vi "Cal_MinimumTriggerStep_from_SweepSpeed.vi"(8 "error in (no error)":errorcluster, 10 "speed":dbl, 11 ".NET Reference in":refnum<k24>) -> (0 "error out":errorcluster, 2 "triggerstep out":dbl, 3 "Reference out":refnum<k24>)   [LabVIEW 2017]
uses:
  LV_IL_Sample/DLL/InstrumentDLL.dll
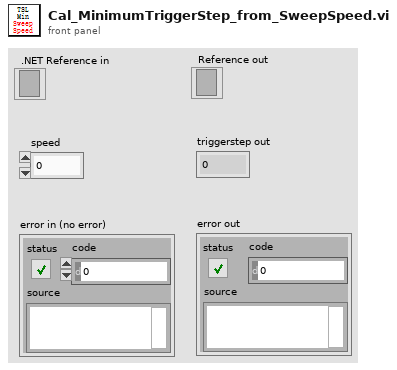
[diagram p1: front panel]
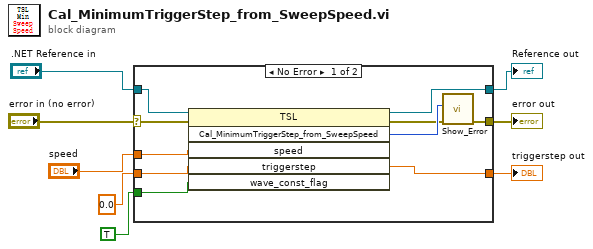
[diagram p0: block diagram]
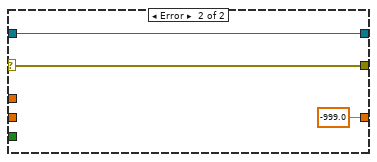
[diagram p2: hidden frame]
diagram:
  n1 = case shown="No Error" "error in (no error)" {
    selector: "error in (no error)" -> [w9 w19]
    tunnel: "speed" -> [w18 _]
    tunnel: ".NET Reference in" -> [w17 w21]
    tunnel: [w16 w21] -> w6
    tunnel: TRUE ("wave_const_flag") -> [w15 _]
    tunnel: 0.0 ("triggerstep") -> [w14 _]
    tunnel: [w12 w19] -> w2
    tunnel: [w10 -999.0 ("triggerstep")] -> w1
    frame No Error {
      n2 = invoke on="调用节点" class="TSL" method="Cal_MinimumTriggerStep_from_SweepSpeed"(reference=w17, error in=w9, "speed"=w18, "triggerstep"=w14, "wave_const_flag"=w15) -> (reference out=w16:refnum<k24>, error out=w11:errorcluster, "Cal_MinimumTriggerStep_from_SweepSpeed"=w13:i32, "triggerstep"=w10:dbl)  [unwired: 1 in, 2 out]
      n3 = call "Show_Error.vi"("error in (no error)"=w11, "Error"=w13) -> ("error out"=w12:errorcluster)  [unwired: 9 in]
    }
    frame Error {
    }
  }
  "Reference out" <- w6
  "error out" <- w2
  "triggerstep out" <- w1
